vi "Periodic Tasks.vi"(8 "error in":errorcluster) -> ()   [LabVIEW 2013]
doc: "This VI runs in parallel to other tasks. It can contain as many user-defined periodic loops as you need. These can carry out PID or other sorts of timed response."
uses:
  <vilib>/Rock Robotics/SystemInterfaces/Utilities/FPGA_UtilitiesLED Source.ctl
  <vilib>/Rock Robotics/SystemInterfaces/Utilities/FPGA_UtilitiesLED State.ctl
  Robot Global Data.vi
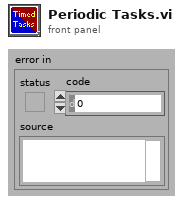
[diagram p1: front panel]
types:
  T1 = typedef "FPGA_UtilitiesLED State.ctl" = enum16{"Off", "On", "Toggle"}
  T2 = typedef "FPGA_UtilitiesLED Source.ctl" = enum16{"User LED", "FPGA LED"}
  T3 = typedef "TeleopInstruction.ctl" = cluster{"cDriveLeft":dbl, "cDriveRight":dbl, "cHalfDrive":bool, "cStraightDrive":bool, "cSonicShifter":bool}
  T4 = typedef "DriveQueueInstruction.ctl" = cluster{"DriveInstruction":T5, "Subsystem":T6, "DriveAction":T7}
  T5 = typedef "DriveInstruction.ctl" = cluster{"cDriveLeft":dbl, "cDriveRight":dbl, "cHalfDrive":bool, "cStraightDrive":bool}
  T6 = typedef "QueueSubsystem.ctl" = enum16{"Drive", "Arm", "Catapult", "Roller"}
  T7 = typedef "DriveAction.ctl" = enum16{"Init", "LinearDrive", "SetValue", "Disable"}
  T8 = typedef "WPI_CompressorDevRef.ctl" = cluster{"DevStatus":errorcluster, "DigitalInputDevRef":T9, "RelayDevRef":T12}
  T9 = typedef "WPI_DigitalInputDevRef.ctl" = cluster{"DevStatus":errorcluster, "DIO Channel":T10, "Digital Module":T11}
  T10 = typedef "FPGA_DIOChannel.ctl" = enum8{"DIO 1", "DIO 2", "DIO 3", "DIO 4", "DIO 5", "DIO 6", "DIO 7", "DIO 8", "DIO 9", "DIO 10", "DIO 11", "DIO 12", "DIO 13", "DIO 14", "Invalid"}
  T11 = typedef "FPGA_TypedefDigitalModule.ctl" = enum16{"Digital Module 1", "Digital Module 2"}
  T12 = typedef "WPI_RelayDevRef.ctl" = cluster{"DevStatus":errorcluster, "Relay Channel":T13, "Digital Module":T11, "Relay Direction":T14}
  T13 = typedef "FPGA_DIORelayChannel.ctl" = enum8{"Relay 1", "Relay 2", "Relay 3", "Relay 4", "Relay 5", "Relay 6", "Relay 7", "Relay 8", "Invalid"}
  T14 = typedef "WPI_RelayDirection.ctl" = enum16{"Both directions", "Forward only", "Reverse only"}
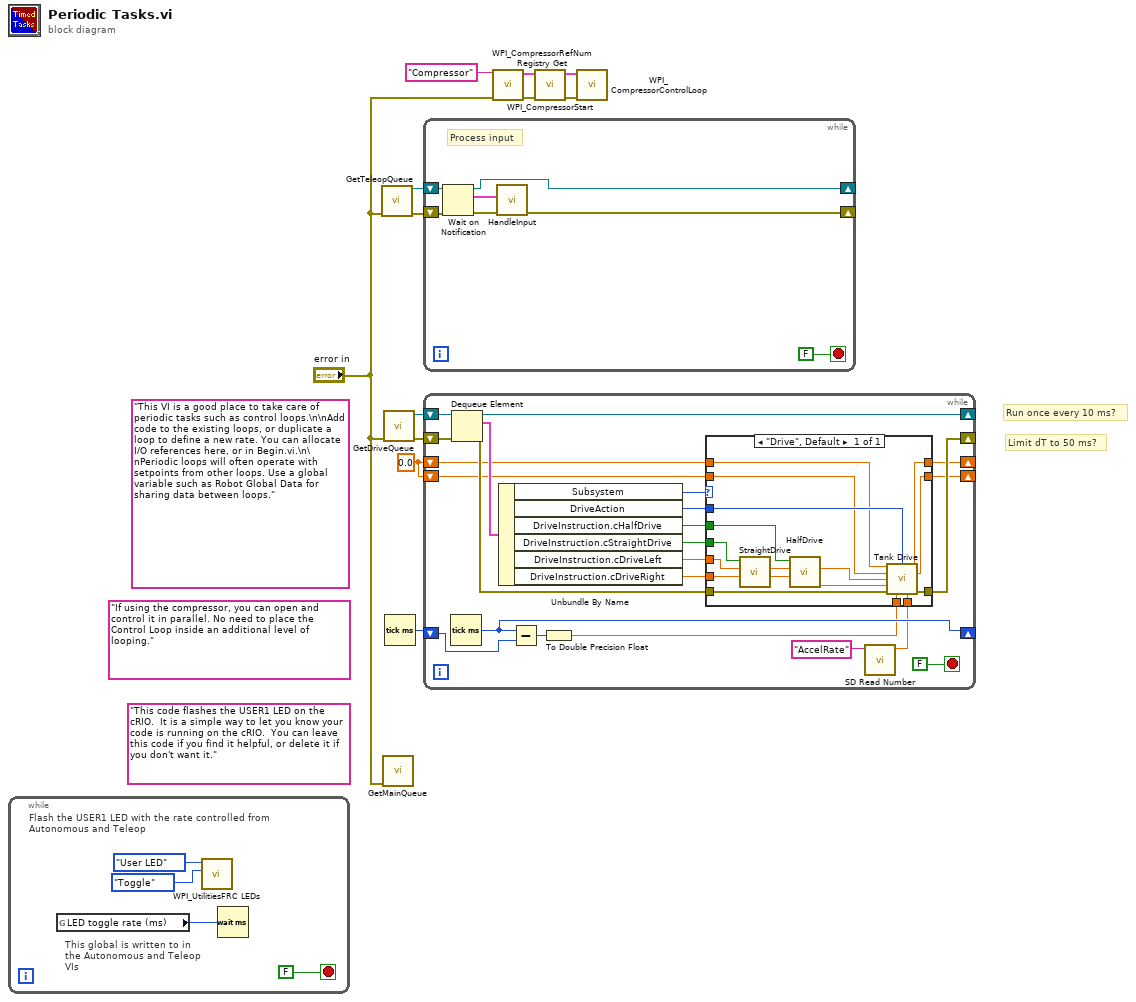
[diagram p0: block diagram]
diagram:
  w1 = 0.0 ("LeftOut")
  (unwired) "If using the compressor, you can open and control it in parallel. No need to place the Control Loop inside an additional level of looping."
  (unwired) "This code flashes the USER1 LED on the cRIO.  It is a simple way to let you know your code is running on the cRIO.  You can leave this code if you find it helpful, or delete it if you don't want it."
  (unwired) "This VI is a good place to take care of periodic tasks such as control loops.\n\nAdd code to the existing loops, or duplicate a loop to define a new rate. You can allocate I/O references here, or in Begin.vi.\n\nPeriodic loops will often operate with setpoints from other loops. Use a global variable such as Robot Global Data for sharing data between loops."
  # "Limit dT to 50 ms?"
  # "Run once every 10 ms?"
  n1 = while {
    stop <- FALSE stop-if-true
    # "This global is written to in the Autonomous and Teleop VIs"
    # "Flash the USER1 LED with the rate controlled from Autonomous and Teleop"
    n2 = global read "Robot Global Data.vi" "LED toggle rate (ms)"() -> (w13:u32)
    n3 = call <vilib>:"WPI_UtilitiesFRC LEDs.vi"("State"=FPGA_UtilitiesLED_State."Toggle", "LED Type"=FPGA_UtilitiesLED_Source."User LED") -> ()  [unwired: 1 in, 9 out]
    n4 = Wait (ms)(milliseconds to wait=w13) -> ()  [unwired: 1 out]
  }
  n5 = call "GetTeleopQueue.vi"("error in (no error)"="error in") -> ("error out"=w7:errorcluster, "notifier out"=w6:refnum<notifier>)  [unwired: 9 in]
  n6 = call "GetMainQueue.vi"("error in (no error)"="error in") -> ()  [unwired: 9 in, 2 out]
  n7 = call "GetDriveQueue.vi"("error in (no error)"="error in") -> ("error out"=w4:errorcluster, "queue out"=w2:refnum<queue>)  [unwired: 9 in]
  n8 = Tick Count (ms)() -> (millisecond timer value=w3:u32)
  n9 = while {
    shift-right: [w20] -> _
    shift-left: w6 -> [w22]
    shift-right: [w18] -> _
    shift-left: w7 -> [w23]
    stop <- FALSE stop-if-true
    # "Process input"
    n10 = Wait on Notification(notifier=w22, error in (no error)=w23) -> (notifier out=w20:refnum<notifier>, notification=w17:T3, error out=w19:errorcluster)  [unwired: 2 in, 1 out]
    n11 = call "HandleInput.vi"("error in (no error)"=w19, "TeleopInstruction"=w17) -> ("error out"=w18:errorcluster)  [unwired: 9 in]
  }
  n12 = while {
    shift-right: [w43] -> _
    shift-left: w4 -> [w45]
    shift-right: [w35] -> _
    shift-left: w2 -> [w36]
    shift-right: [w41] -> _
    shift-left: w3 -> [w42]
    shift-right: [w26] -> _
    shift-left: w1 -> [w25]
    shift-right: [w27] -> _
    shift-left: w1 -> [w24]
    stop <- FALSE stop-if-true
    n13 = Tick Count (ms)() -> (millisecond timer value=w41:u32)
    n14 = Dequeue Element(queue=w36, error in (no error)=w45) -> (queue out=w35:refnum<queue>, element=w34:T4, error out=w44:errorcluster)  [unwired: 1 in, 1 out]
    n15 = Unbundle By Name(w34) -> ("Subsystem"=w33:T6, "DriveAction"=w32:T7, "DriveInstruction.cHalfDrive"=w31:bool, "DriveInstruction.cStraightDrive"=w30:bool, "DriveInstruction.cDriveLeft"=w29:dbl, "DriveInstruction.cDriveRight"=w28:dbl)
    n16 = Subtract(x=w41, y=w42) -> (x-y=w37:u32)
    n17 = To Double Precision Float(number=w37) -> (double precision float=w40:dbl)
    n18 = call <vilib>:"SD Read Number.vi"("Name"="AccelRate") -> ("Numeric"=w38:dbl)  [unwired: 8 in, 2 out]
    n19 = case shown="\"Drive\", Default" w33 {
      tunnel: w44 -> [w59]
      tunnel: [w58] -> w43
      tunnel: w40 -> [w57]
      tunnel: w38 -> [w56]
      tunnel: w32 -> [w55]
      tunnel: w31 -> [w53]
      tunnel: w30 -> [w54]
      tunnel: w29 -> [w52]
      tunnel: w28 -> [w51]
      tunnel: [w50] -> w26
      tunnel: [w49] -> w27
      tunnel: w25 -> [w48]
      tunnel: w24 -> [w47]
      frame "Drive", Default {
        n20 = call "StraightDrive.vi"("RightDrive in"=w51, "LeftDrive in"=w52, "StraightDrive"=w54) -> ("RightDrive out"=w62:dbl, "LeftDrive out"=w63:dbl)  [unwired: 7 in]
        n21 = call "HalfDrive.vi"("RightDrive in"=w62, "LeftDrive in"=w63, "HalfDrive"=w53) -> ("RightDrive out"=w60:dbl, "LeftDrive out"=w61:dbl)  [unwired: 7 in]
        n22 = call "Tank Drive.vi"("LeftActual"=w48, "DriveAction"=w55, "Right Actual"=w47, "LeftDesired"=w61, "RightDesired"=w60, "error in (no error)"=w59, "LoopTime"=w57, "AccelRate"=w56) -> ("LeftOut"=w50:dbl, "RightOut"=w49:dbl, "error out"=w58:errorcluster)  [unwired: 5 in]
      }
    }
  }
  n23 = call <vilib>:"WPI_CompressorRefNum Registry Get.vi"("error in (no error)"="error in", "refnum name"="Compressor") -> ("error out"=w9:errorcluster, "CompressorDevRef"=w12:T8)  [unwired: 8 in]
  n24 = call <vilib>:"WPI_CompressorStart.vi"("error in (no error)"=w9, "CompressorDevRef"=w12) -> ("error out"=w8:errorcluster, "CompressorDevRef"=w11:T8)  [unwired: 8 in]
  n25 = call <vilib>:"WPI_CompressorControlLoop.vi"("error in (no error)"=w8, "CompressorDevRef"=w11) -> ()  [unwired: 10 in]
